vi "Symbol to DataLen.vi"(1 "QAM Comparison":enum16{"MT Modulate", "Homebrew"}(ring), 2 "Number of Symbols":i32, 3 "QAM Complexity":T1(ring)) -> (0 "DataLen":i32)   [LabVIEW 2018]
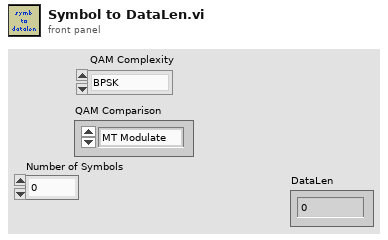
[diagram p1: front panel]
types:
  T1 = enum16{"BPSK", "QPSK", "16-QAM", "64-QAM", "256-QAM"}
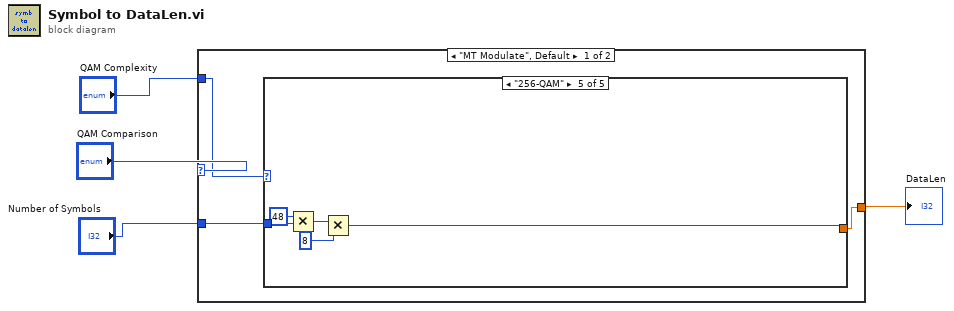
[diagram p0: block diagram]
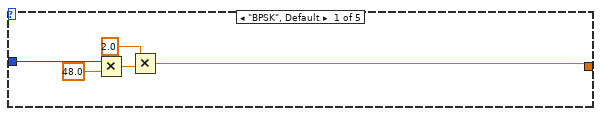
[diagram p2: hidden frame]
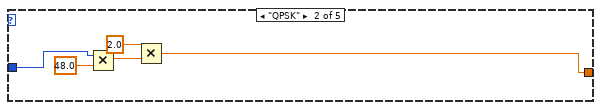
[diagram p3: hidden frame]
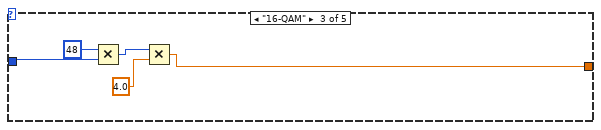
[diagram p4: hidden frame]
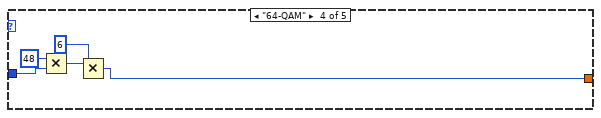
[diagram p5: hidden frame]
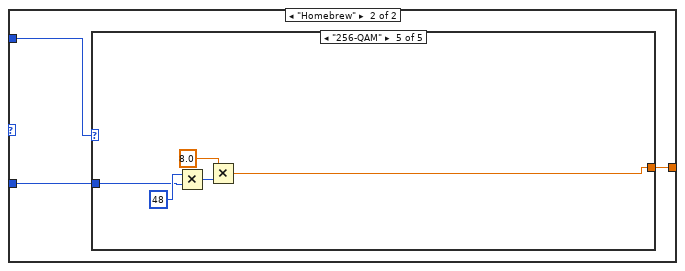
[diagram p6: hidden frame]
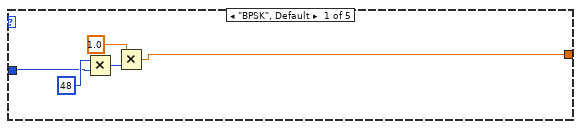
[diagram p7: hidden frame]
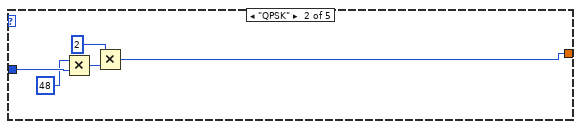
[diagram p8: hidden frame]
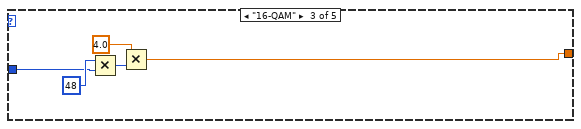
[diagram p9: hidden frame]
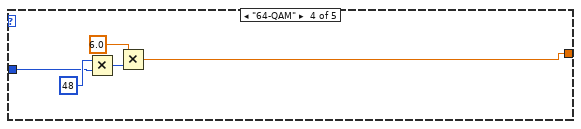
[diagram p10: hidden frame]
diagram:
  n1 = case shown="\"MT Modulate\", Default" "QAM Comparison" {
    tunnel: "QAM Complexity" -> [w7 w35]
    tunnel: "Number of Symbols" -> [w6 w34]
    tunnel: [w5 w33] -> w1
    frame "MT Modulate", Default {
      n2 = case shown="\"256-QAM\"" w7 {
        tunnel: w6 -> [w12 w16 w22 w27 w32]
        tunnel: [w9 w14 w18 w23 w28] -> w5
        frame "BPSK", Default {
          n3 = Multiply(x=w12, y=48.0) -> (x*y=w10:dbl)
          n4 = Multiply(x=2.0, y=w10) -> (x*y=w9:dbl)
        }
        frame "QPSK" {
          n5 = Multiply(x=w16, y=48.0) -> (x*y=w15:dbl)
          n6 = Multiply(x=2.0, y=w15) -> (x*y=w14:dbl)
        }
        frame "16-QAM" {
          n7 = Multiply(x=48, y=w22) -> (x*y=w20:i32)
          n8 = Multiply(x=w20, y=4.0) -> (x*y=w18:dbl)
        }
        frame "64-QAM" {
          n9 = Multiply(x=48, y=w27) -> (x*y=w25:i32)
          n10 = Multiply(x=w25, y=6) -> (x*y=w23:i32)
        }
        frame "256-QAM" {
          n11 = Multiply(x=48, y=w32) -> (x*y=w30:i32)
          n12 = Multiply(x=w30, y=8) -> (x*y=w28:i32)
        }
      }
    }
    frame "Homebrew" {
      n13 = case shown="\"256-QAM\"" w35 {
        tunnel: w34 -> [w37 w45 w47 w52 w57]
        tunnel: [w36 w41 w46 w51 w56] -> w33
        frame "BPSK", Default {
          n14 = Multiply(x=48 ("y"), y=w37) -> (x*y=w39:i32)
          n15 = Multiply(x=1.0, y=w39) -> (x*y=w36:dbl)
        }
        frame "QPSK" {
          n16 = Multiply(x=48 ("y"), y=w45) -> (x*y=w43:i32)
          n17 = Multiply(x=2, y=w43) -> (x*y=w41:i32)
        }
        frame "16-QAM" {
          n18 = Multiply(x=48 ("y"), y=w47) -> (x*y=w49:i32)
          n19 = Multiply(x=4.0, y=w49) -> (x*y=w46:dbl)
        }
        frame "64-QAM" {
          n20 = Multiply(x=48 ("y"), y=w52) -> (x*y=w54:i32)
          n21 = Multiply(x=6.0, y=w54) -> (x*y=w51:dbl)
        }
        frame "256-QAM" {
          n22 = Multiply(x=48 ("y"), y=w57) -> (x*y=w59:i32)
          n23 = Multiply(x=8.0, y=w59) -> (x*y=w56:dbl)
        }
      }
    }
  }
  "DataLen" <- w1
